vi "circ_ap && forvard.vi"() -> ()   [LabVIEW 2012, in "LightPipes.lvlib"]
uses:
  LightPipes.lvlib
panel:
  in  "distance":dbl=1.0
  out "Field":cluster{"n_grid":i32, "size":dbl, "lambda":dbl}
  # "Beam Characteristic"
  # "Circular Apprature"
  # "Forward"
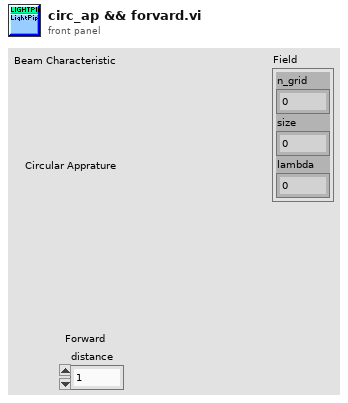
[diagram p1: front panel]
types:
  T1 = cluster{"n_grid":i32, "@dummy control@":i8, "@dummy control@":i8, "@dummy control@":i8, "@dummy control@":i8, "size":dbl, "lambda":dbl, "int1":i32, "int2":i32, "int3":i32, "@dummy control@":i8, "@dummy control@":i8, "@dummy control@":i8, "@dummy control@":i8, "double1":dbl, "double2":dbl, "double3":dbl, "real":u32, "imaginary":u32}
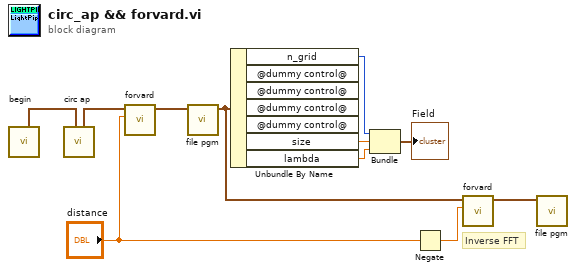
[diagram p0: block diagram]
diagram:
  # "Inverse FFT"
  n1 = call "begin.vi"() -> ("field out"=w7:T1)  [unwired: 11 in]
  n2 = call "circ ap.vi"("field"=w7) -> ("field out"=w6:T1)  [unwired: 10 in]
  n3 = call "forvard.vi"("distance"="distance", "field"=w6) -> ("field out"=w3:T1)  [unwired: 9 in]
  n4 = call "file pgm.vi"("field"=w3) -> ("field out"=w2:T1)  [unwired: 9 in, 1 out]
  n5 = Unbundle By Name(w2) -> ("n_grid"=w8:i32, "size"=w9:dbl, "lambda"=w10:dbl)  [unwired: 4 out]
  n6 = Bundle("n_grid"=w8, "size"=w9, "lambda"=w10) -> (→"Field":cluster{"n_grid":i32, "size":dbl, "lambda":dbl})  [unwired: 1 in]
  n7 = Negate(x="distance") -> (-x=w4:dbl)
  n8 = call "forvard.vi"("distance"=w4, "field"=w2) -> ("field out"=w1:T1)  [unwired: 9 in]
  n9 = call "file pgm.vi"("field"=w1) -> ()  [unwired: 9 in, 2 out]
